vi "Instrument Types.vi"(8 "error in (no error)":errorcluster, 11 "ExampleInstrument in":refnum<class "LevyLab Instrument.lvclass">) -> (0 "error out":errorcluster, 3 "ExampleInstrument out":refnum<class "LevyLab Instrument.lvclass">)   [LabVIEW 2016, in "LevyLab Instrument.lvclass"]
uses:
  LevyLab Instrument.lvclass
  Instrument Types/Cryostat/Instrument.Cryostat.lvclass
  Instrument Types/VSource/Instrument.VSource.lvclass
  Instrument Types/VNA/Instrument.VNA.lvclass
  Instrument Types/CBridge/Instrument.CBridge.lvclass
  Instrument Types/Strain/Instrument.Strain.lvclass
  Instrument Types/Optical Delay Line/Instrument.OpticalDelayLine.lvclass
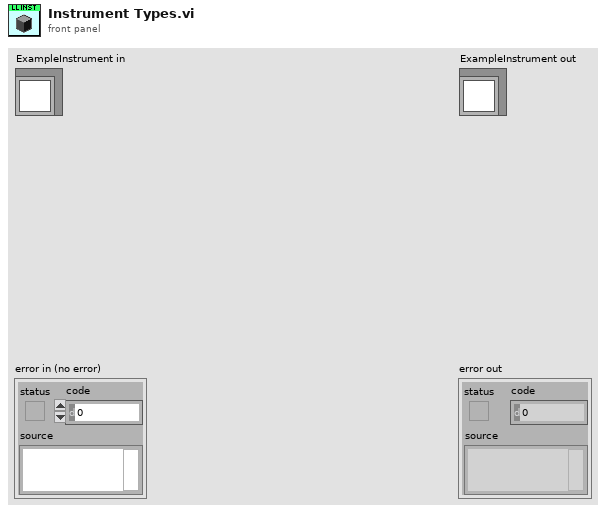
[diagram p1: front panel]
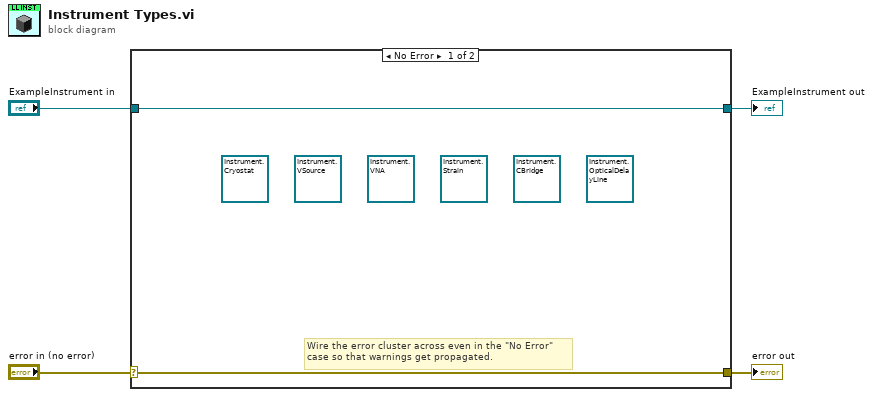
[diagram p0: block diagram]
diagram:
  n1 = case shown="No Error" "error in (no error)" {
    selector: "error in (no error)" -> [w5 w8]
    tunnel: [w5 w8] -> w3
    tunnel: [w6 w7] -> w1
    tunnel: "ExampleInstrument in" -> [w6 w7]
    frame No Error {
      (unwired) refnum<class "Instrument.OpticalDelayLine.lvclass"> refnum ("Instrument.OpticalDelayLine.lvclass")
      (unwired) refnum<class "Instrument.Strain.lvclass"> refnum ("Instrument.Strain.lvclass")
      (unwired) refnum<class "Instrument.CBridge.lvclass"> refnum ("Instrument.CBridge.lvclass")
      (unwired) refnum<class "Instrument.VNA.lvclass"> refnum ("Instrument.VNA.lvclass")
      (unwired) refnum<class "Instrument.VSource.lvclass"> refnum ("Instrument.VSource.lvclass")
      (unwired) refnum<class "Instrument.Cryostat.lvclass"> refnum ("Instrument.Cryostat.lvclass")
      # "Wire the error cluster across even in the \"No Error\"\ncase so that warnings get propagated."
    }
    frame Error {
    }
  }
  "error out" <- w3
  "ExampleInstrument out" <- w1
